vi "minus.vi"(1 "MINUS":bool, 2 "INPUT":T2) -> (0 "OUTPUT":T1)   [LabVIEW 2013]
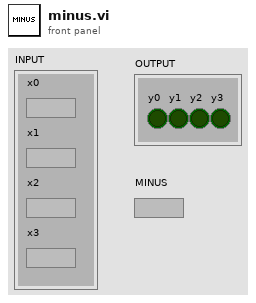
[diagram p1: front panel]
types:
  T1 = cluster{"y0":bool, "y1":bool, "y2":bool, "y3":bool}
  T2 = cluster{"x0":bool, "x1":bool, "x2":bool, "x3":bool}
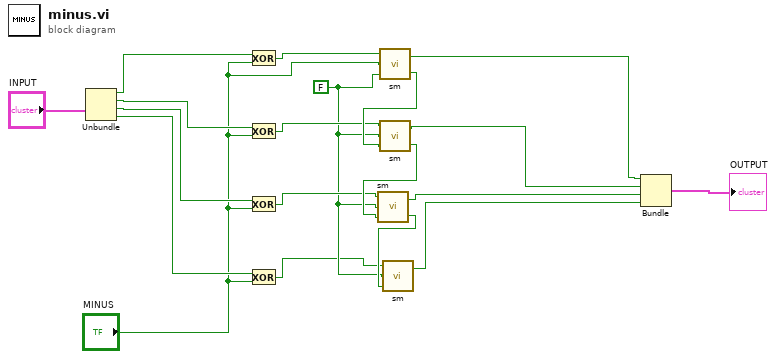
[diagram p0: block diagram]
diagram:
  w3 = FALSE
  n1 = Unbundle("INPUT") -> ("x0"=w18:bool, "x1"=w15:bool, "x2"=w16:bool, "x3"=w17:bool)
  n2 = Exclusive Or(1:"MINUS", 2:w18) -> (0:w13:bool)
  n3 = Exclusive Or(1:"MINUS", 2:w15) -> (0:w9:bool)
  n4 = Exclusive Or(1:"MINUS", 2:w16) -> (0:w6:bool)
  n5 = Exclusive Or(1:"MINUS", 2:w17) -> (0:w2:bool)
  n6 = call "sm.vi"("c"=w3, "b"="MINUS", "a"=w13) -> ("C"=w10:bool, "S"=w11:bool)
  n7 = call "sm.vi"("c"=w10, "b"=w3, "a"=w9) -> ("C"=w7:bool, "S"=w8:bool)
  n8 = call "sm.vi"("c"=w7, "b"=w3, "a"=w6) -> ("C"=w4:bool, "S"=w5:bool)
  n9 = call "sm.vi"("c"=w4, "b"=w3, "a"=w2) -> ("S"=w1:bool)  [unwired: 1 out]
  n10 = Bundle("S"=w11, "S"=w8, "S"=w5, "S"=w1) -> (→"OUTPUT":cluster{"S":bool, "S":bool, "S":bool, "S":bool})  [unwired: 1 in]
